vi "Auto Shooter Wheels.vi"(8 "error in (no error)":errorcluster, 11 "Robot Commands":T1) -> (0 "error out":errorcluster)   [LabVIEW 2014]
uses:
  SubSystems/Joystick/Robot Commands.ctl
  Global Variables/Global Variables.vi
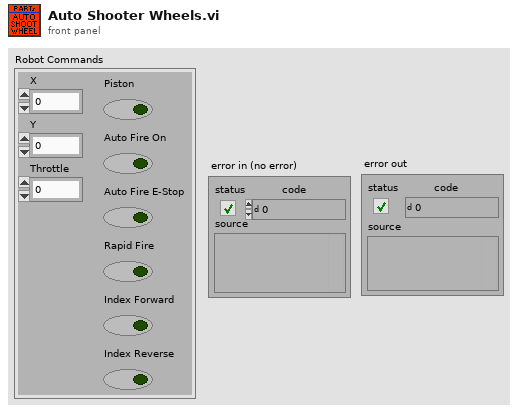
[diagram p1: front panel]
types:
  T1 = typedef "Robot Commands.ctl" = cluster{"X":dbl, "Y ":dbl, "Throttle":dbl, "Piston":bool, "Auto Fire On":bool, "Auto Fire E-Stop":bool, "Rapid Fire":bool, "Index Forward":bool, "Index Reverse ":bool}
  T2 = typedef "WPI_MotorControlDeviceRef.ctl" = cluster{"DeviceStatus":errorcluster, "Type":T3, "PWM":cluster{"Controller":T4, "PWM Channel":T5, "DeadBand":T6}, "CAN":cluster{"Device Number":u8, "Control Mode":T7, "Semaphore":T8, "Max Vout":dbl, "TalonSRX Control Mode":T9}, "Invert":bool, "TransformRef":T10, "InvTransformRef":T10}
  T3 = typedef "WPI_MotorControlType.ctl" = enum16{"PWM", "CAN", "CANTalonSRX"}
  T4 = typedef "FPGA_TypedefDigitalModule.ctl" = enum16{"Controller 1"}
  T5 = typedef "FPGA_DIOPWMChannel.ctl" = enum8{"PWM 0", "PWM 1", "PWM 2", "PWM 3", "PWM 4", "PWM 5", "PWM 6", "PWM 7", "PWM 8", "PWM 9", "PWM MXP 0", "PWM MXP 1", "PWM MXP 2", "PWM MXP 3", "PWM MXP 4", "PWM MXP 5", "PWM MXP 6", "PWM MXP 7", "PWM MXP 8", "PWM MXP 9", "Invalid"}
  T6 = typedef "WPI_PWMDeadband.ctl" = cluster{"Name":string, "maxPositivePwm":i32, "minPositivePwm":i32, "centerPwm":i32, "maxNegativePwm":i32, "minNegativePwm":i32, "angularRange":u16}
  T7 = typedef "WPI_CANJaguar_ControlMode.ctl" = enum8{"Percent VBus", "Current", "Speed", "Position", "Voltage"}
  T8 = typedef "Semaphore RefNum" = refnum<k1>
  T9 = typedef "WPI_CANTalonSRX_APIControlMode.ctl" = enum8{"Percent VBus", "Speed", "Position", "Slave", "Unchanged / Invalid"}
  T10 = typedef "WPI_PWMTransform_ConPane.ctl" = refnum<vi>
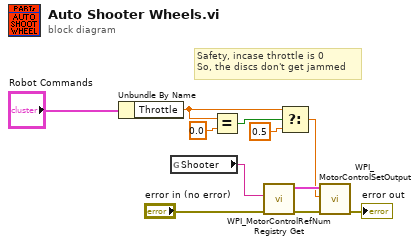
[diagram p0: block diagram]
diagram:
  # "Safety, incase throttle is 0\nSo, the discs don't get jammed"
  n1 = Unbundle By Name("Robot Commands") -> ("Throttle"=w4:dbl)
  n2 = global read "Global Variables.vi" "Shooter"() -> (w8:string)
  n3 = Equal?(x=w4, y=0.0) -> (x = y?=w2:bool)
  n4 = call <vilib>:"WPI_MotorControlRefNum Registry Get.vi"("error in (no error)"="error in (no error)", "refnum name"=w8) -> ("error out"=w10:errorcluster, "MotorControlDevRef"=w9:T2)  [unwired: 8 in]
  n5 = Select(t=w4, s=w2, f=0.5) -> (s? t:f=w5:dbl)
  n6 = call <vilib>:"WPI_MotorControlSetOutput.vi"("error in (no error)"=w10, "Output"=w5, "MotorControlDevRef"=w9) -> ("error out"=→"error out":errorcluster)  [unwired: 6 in, 2 out]
